vi "From Datum Array.vi"(0 "Data":T1(array[cluster])) -> (2 "Map":refnum<class "Map.lvclass">)   [LabVIEW 2018]
uses:
  Map.lvclass
  D:/Users/cfield/Code/Field R&D Services/Mustache/LabVIEW/trunk/src/Toolkit/Data/Datum/Datum.lvclass
  Datum/Datum.lvclass
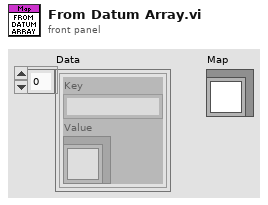
[diagram p1: front panel]
types:
  T1 = cluster{"Key":string, "Value":refnum<class "Datum.lvclass">}[]
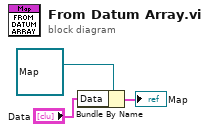
[diagram p0: block diagram]
diagram:
  n1 = Bundle By Name(cluster=refnum<class "Map.lvclass"> refnum ("Toolkit.lvlib:Data.lvlib:Map.lvclass"), "Data"="Data") -> (→"Map":cluster{})
